vi "FGV IN.vi"(0 "DI":T5, 5 "Analog Eingänge":T3, 7 "TC Eingänge":T1, 9 "Fühler Bruch TC":T2, 11 "Fühler Bruch AI":T4, 12 "Aktion":T6) -> (4 "DI":T5, 6 "Analog Eingänge":T3, 8 "TC Eingänge":T1, 10 "Fühler Bruch TC":T2, 15 "Fühler Bruch AI":T4)   [LabVIEW 2020, in "Verwaltung - cRIO.lvlib"]
uses:
  Verwaltung - cRIO.lvlib
  FGV IN Aktionen.ctl
  Digital Eingaenge 0-15.ctl
  Fuehler Bruch AI.ctl
  Analog Eingaenge.ctl
  Fuehler Bruch TC.ctl
  TC Eingaenge.ctl
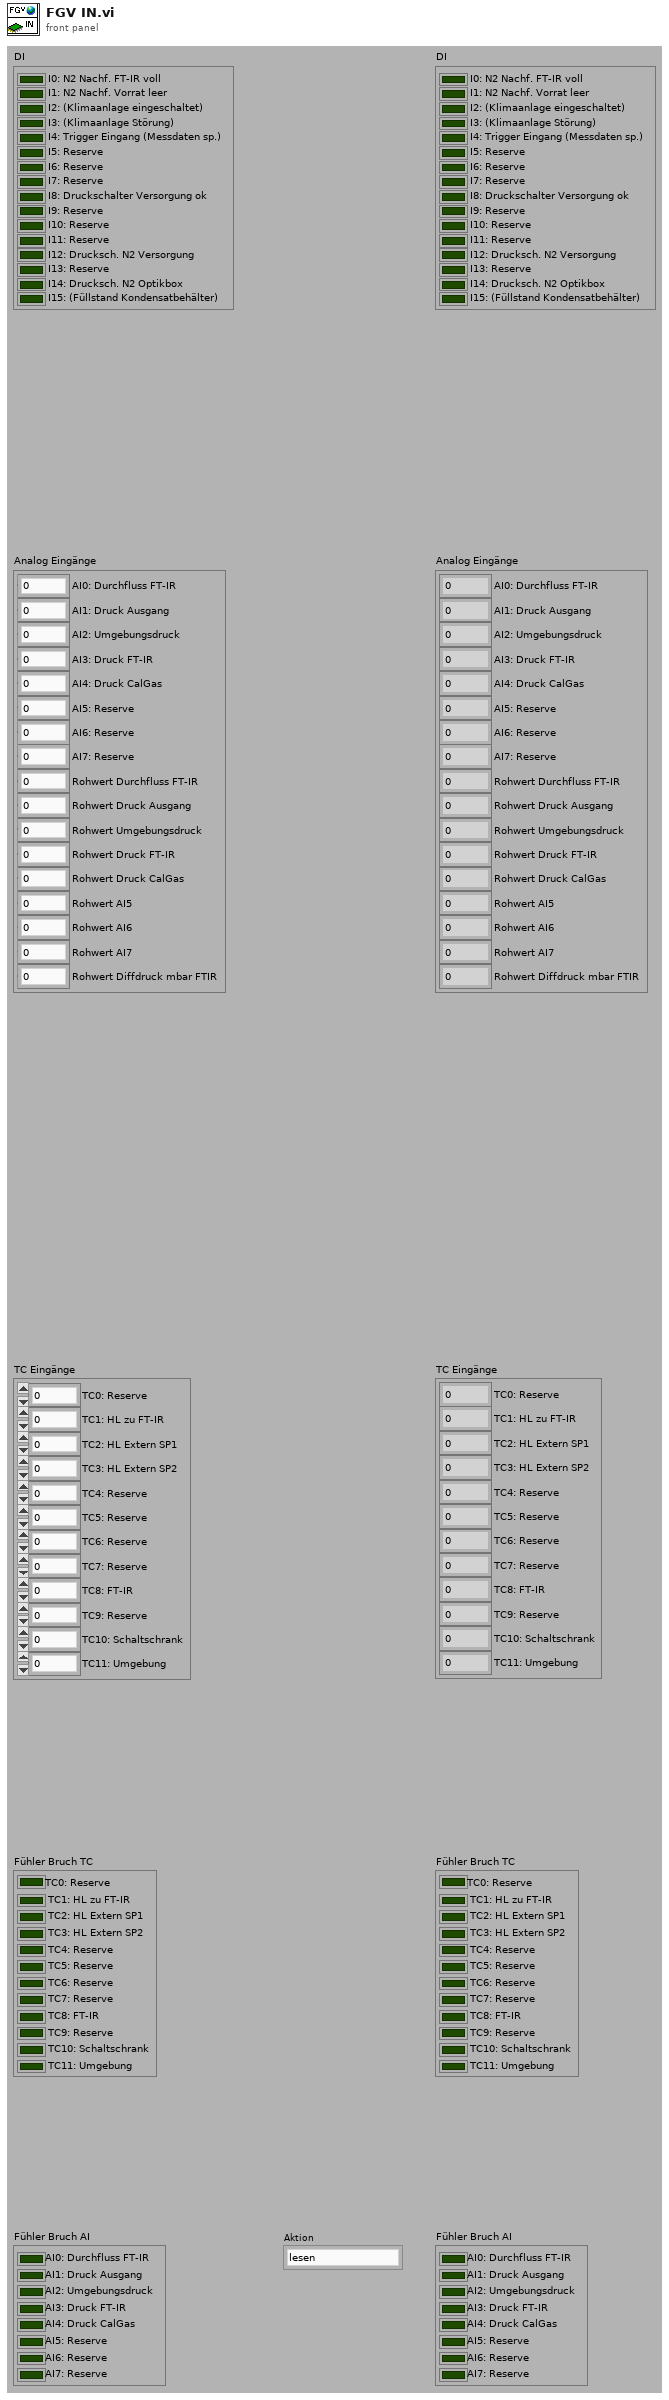
[diagram p1: front panel]
types:
  T1 = typedef "Verwaltung - cRIO.lvlib/TC Eingaenge.ctl" = cluster{"TC0: Reserve":sgl, "TC1: HL zu FT-IR":sgl, "TC2: HL Extern SP1":sgl, "TC3: HL Extern SP2":sgl, "TC4: Reserve":sgl, "TC5: Reserve":sgl, "TC6: Reserve":sgl, "TC7: Reserve":sgl, "TC8: FT-IR":sgl, "TC9: Reserve":sgl, "TC10: Schaltschrank":sgl, "TC11: Umgebung":sgl}
  T2 = typedef "Verwaltung - cRIO.lvlib/Fuehler Bruch TC.ctl" = cluster{"TC0: Reserve":bool, "TC1: HL zu FT-IR":bool, "TC2: HL Extern SP1":bool, "TC3: HL Extern SP2":bool, "TC4: Reserve":bool, "TC5: Reserve":bool, "TC6: Reserve":bool, "TC7: Reserve":bool, "TC8: FT-IR":bool, "TC9: Reserve":bool, "TC10: Schaltschrank":bool, "TC11: Umgebung":bool}
  T3 = typedef "Verwaltung - cRIO.lvlib/Analog Eingaenge.ctl" = cluster{"AI0: Durchfluss FT-IR":sgl, "AI1: Druck Ausgang":sgl, "AI2: Umgebungsdruck":sgl, "AI3: Druck FT-IR":sgl, "AI4: Druck CalGas":sgl, "AI5: Reserve":sgl, "AI6: Reserve":sgl, "AI7: Reserve":sgl, "Rohwert Durchfluss FT-IR":sgl, "Rohwert Druck Ausgang":sgl, "Rohwert Umgebungsdruck":sgl, "Rohwert Druck FT-IR":sgl, "Rohwert Druck CalGas":sgl, "Rohwert AI5":sgl, "Rohwert AI6":sgl, "Rohwert AI7":sgl, "Rohwert Diffdruck mbar FTIR":sgl}
  T4 = typedef "Verwaltung - cRIO.lvlib/Fuehler Bruch AI.ctl" = cluster{"AI0: Durchfluss FT-IR":bool, "AI1: Druck Ausgang":bool, "AI2: Umgebungsdruck":bool, "AI3: Druck FT-IR":bool, "AI4: Druck CalGas":bool, "AI5: Reserve":bool, "AI6: Reserve":bool, "AI7: Reserve":bool}
  T5 = typedef "Verwaltung - cRIO.lvlib/Digital Eingaenge 0-15.ctl" = cluster{"I0: N2 Nachf. FT-IR voll":bool, "I1: N2 Nachf. Vorrat leer":bool, "I2: (Klimaanlage eingeschaltet)":bool, "I3: (Klimaanlage Störung)":bool, "I4: Trigger Eingang (Messdaten sp.)":bool, "I5: Reserve":bool, "I6: Reserve":bool, "I7: Reserve":bool, "I8: Druckschalter Versorgung ok":bool, "I9: Reserve":bool, "I10: Reserve":bool, "I11: Reserve":bool, "I12: Drucksch. N2 Versorgung":bool, "I13: Reserve":bool, "I14: Drucksch. N2 Optikbox":bool, "I15: (Füllstand Kondensatbehälter)":bool}
  T6 = typedef "Verwaltung - cRIO.lvlib/FGV IN Aktionen.ctl" = enum16{"lesen", "DI", "AI", "Fühler Br.", "TC", "Fühler Br. TC"}
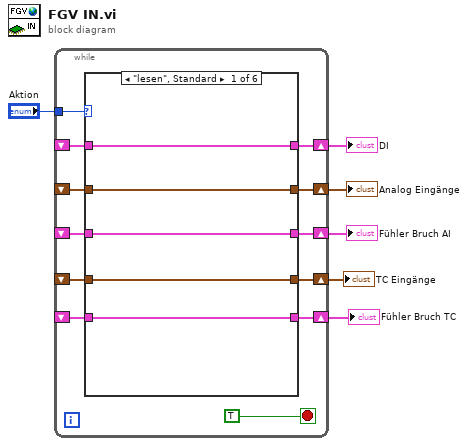
[diagram p0: block diagram]
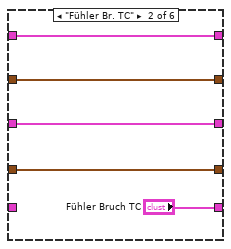
[diagram p2: hidden frame]
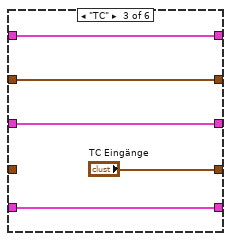
[diagram p3: hidden frame]
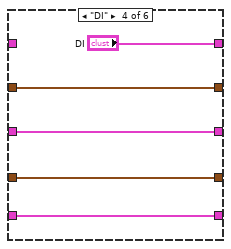
[diagram p4: hidden frame]
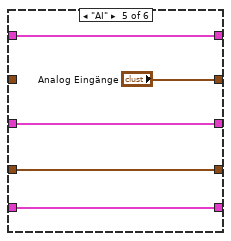
[diagram p5: hidden frame]
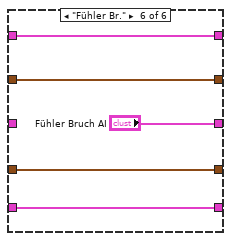
[diagram p6: hidden frame]
diagram:
  n1 = while {
    tunnel: "Aktion" -> [w17]
    shift-right: [w16] -> w5
    shift-left: _ -> [w15]
    shift-right: [w11] -> w4
    shift-left: _ -> [w14]
    shift-right: [w12] -> w3
    shift-left: _ -> [w13]
    shift-right: [w10] -> w2
    shift-left: _ -> [w9]
    shift-right: [w8] -> w1
    shift-left: _ -> [w7]
    stop <- TRUE stop-if-true
    n2 = case shown="\"lesen\", Standard" w17 {
      tunnel: [w23 w28 w33 "DI" w43 w48] -> w16
      tunnel: w15 -> [w23 w28 w33 _ w43 w48]
      tunnel: w14 -> [w22 w27 w32 w37 _ w47]
      tunnel: w13 -> [w21 w26 w31 w38 w42 _]
      tunnel: [w21 w26 w31 w38 w42 "Fühler Bruch AI"] -> w12
      tunnel: [w22 w27 w32 w37 "Analog Eingänge" w47] -> w11
      tunnel: [w20 w25 "TC Eingänge" w35 w40 w45] -> w10
      tunnel: w9 -> [w20 w25 _ w35 w40 w45]
      tunnel: [w19 "Fühler Bruch TC" w29 w34 w39 w44] -> w8
      tunnel: w7 -> [w19 _ w29 w34 w39 w44]
      frame "lesen", Default {
      }
      frame "Fühler Br. TC" {
      }
      frame "TC" {
      }
      frame "DI" {
      }
      frame "AI" {
      }
      frame "Fühler Br." {
      }
    }
  }
  "DI" <- w5
  "Fühler Bruch AI" <- w3
  "Analog Eingänge" <- w4
  "Fühler Bruch TC" <- w1
  "TC Eingänge" <- w2
